vi "keyboard_monitor.vi"() -> ()   [LabVIEW 2019]
uses:
  <vilib>/Utility/inputDevices.llb/keyboardAcquire.vi
panel:
  out "error out":errorcluster
  out "handle out":i32
  in  "step":dbl
  in  "error in (no error)":errorcluster
  in  "handle in":i32
  in  "Up":bool
  in  "Down":bool
  in  "^":bool
  in  "v":bool
  in  ">":bool
  in  "<":bool
  out "x":dbl
  out "y":dbl
  out "z":dbl
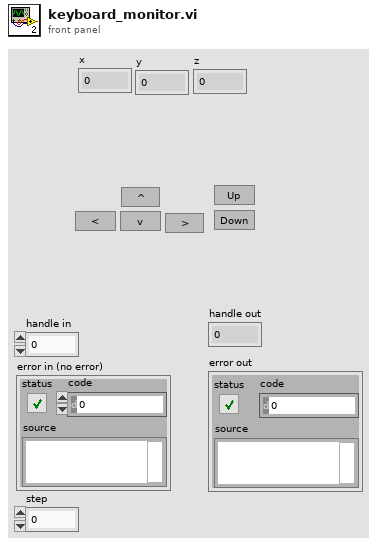
[diagram p1: front panel]
types:
  T1 = enum16{"0", "1", "2", "3", "4", "5", "6", "7", "8", "9", "A", "B", "C", "D", "E", "F", "G", "H", "I", "J", "K", "L", "M", "N", "O", "P", "Q", "R", "S", "T", "U", "V", "W", "X", "Y", "Z", "F1", "F2", "F3", "F4", "F5", "F6", "F7", "F8", "F9", "F10", "F11", "F12", "F13", "F14", "F15", "ADD", "BACK", "BACKSLASH", "CAPITAL", "COMMA", "DECIMAL", "DELETE", "DIVIDE", "DOWN", "END", "EQUALS", "ESCAPE", "GRAVE (`)", "HOME", "INSERT", "LBRACKET", "LCONTROL", "LEFT", "L ALT", "LSHIFT", "LWIN", "MINUS", "MULTIPLY", "NEXT", "NUMLOCK", "NUMPAD_0", "NUMPAD_1", "NUMPAD_2", "NUMPAD_3", "NUMPAD_4", "NUMPAD_5", "NUMPAD_6", "NUMPAD_7", "NUMPAD_8", "NUMPAD_9", "PAUSE", "PERIOD", "PRIOR (PG UP)", "RBRACKET", "RCONTROL", "RETURN", "RIGHT", "R ALT", "RSHIFT", "RWIN", "SCROLL", "SEMICOLON", "SLASH", "SPACE", "SUBTRACT", "TAB", "UP", "ENTER (num pad)", "' (quote)"}[]
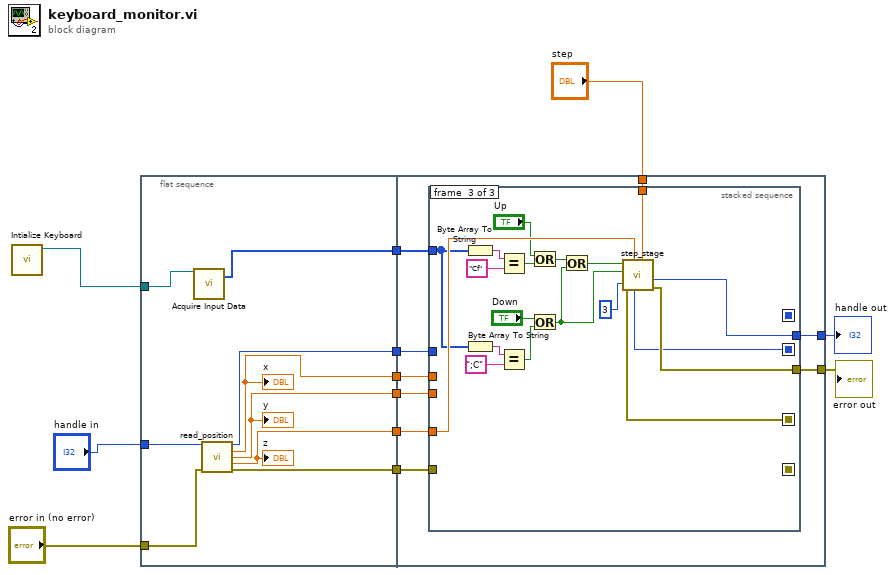
[diagram p0: block diagram]
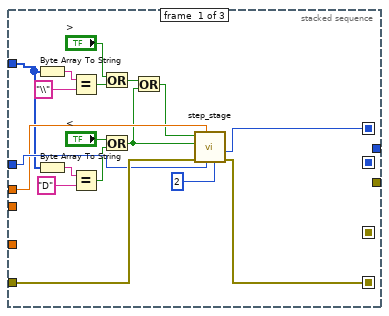
[diagram p2: hidden frame]
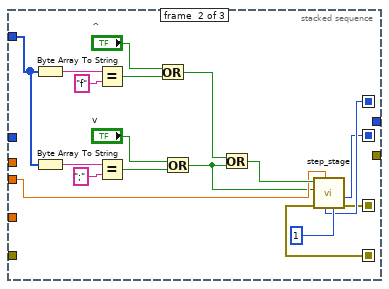
[diagram p3: hidden frame]
diagram:
  n1 = call <vilib>:"Intialize Keyboard.vi"() -> ("device ID"=w7:refnum<k1>)  [unwired: 1 in, 10 out]
  n2 = flat-sequence {
    tunnel: [w21] -> w12
    tunnel: [w20] -> w11
    tunnel: [w19] -> w10
    tunnel: [w18] -> w9
    tunnel: [w17] -> w8
    tunnel: w7 -> [w16]
    tunnel: [w15] -> w6
    tunnel: "handle in" -> [w14]
    tunnel: "error in (no error)" -> [w13]
    tunnel: w12 -> [w30]
    tunnel: w11 -> [w29]
    tunnel: w10 -> [w28]
    tunnel: w9 -> [w27]
    tunnel: w8 -> [w26]
    tunnel: [w25] -> w1
    tunnel: [w24] -> w2
    tunnel: w6 -> [w23]
    tunnel: "step" -> [w22]
    frame #0 {
      n3 = call-poly <vilib>:"Acquire Input Data.vi"("device ID"=w16) -> ("keys pressed"=w15:T1)  [unwired: 1 in, 17 out]
      n4 = call "read_position.vi"("handle in"=w14, "error in (no error)"=w13) -> ("handle out"=w20:i32, "x"=w19:dbl, "y"=w18:dbl, "z"=w17:dbl, "error out"=w21:errorcluster)  [unwired: 9 in]
      "x" <- w19
      "y" <- w18
      "z" <- w17
    }
    frame #1 {
      n5 = stacked-sequence {
        seq-local: [w44 _ _] -> [_ w63 _]
        seq-local: [w43 _ _] -> [_ w62 _]
        seq-local: [_ w60 _] -> [_ _ w81]
        seq-local: [_ w61 _] -> [_ _ w80]
        tunnel: w30 -> [w48 _ _]
        tunnel: w29 -> [w47 _ _]
        tunnel: w28 -> [w45 _ _]
        tunnel: w27 -> [_ w64 _]
        tunnel: w26 -> [_ _ w84]
        tunnel: [_ _ w82] -> w25
        tunnel: [_ _ w83] -> w24
        tunnel: w23 -> [w31 w49 w68]
        tunnel: w22 -> [_ _ w67]
        frame #0 {
          n6 = Byte Array To String(unsigned byte array=w31) -> (string=w42:string)
          n7 = Byte Array To String(unsigned byte array=w31) -> (string=w40:string)
          n8 = Equal?(x=w42, y="\\") -> (x = y?=w38:bool)
          n9 = Equal?(x=w40, y="D") -> (x = y?=w37:bool)
          n10 = Or(x=">", y=w38) -> (x .or. y?=w36:bool)
          n11 = Or(x="<", y=w37) -> (x .or. y?=w33:bool)
          n12 = Or(x=w36, y=w33) -> (x .or. y?=w32:bool)
          n13 = call "step_stage.vi"("axis"=u32 2, "handle"=w47, "position"=w45, "error in"=w48, "+/-"=w33, "move"=w32) -> ("error out"=w43:errorcluster, "handle out"=w44:i32)  [unwired: 4 in]
        }
        frame #1 {
          n14 = Byte Array To String(unsigned byte array=w49) -> (string=w59:string)
          n15 = Byte Array To String(unsigned byte array=w49) -> (string=w57:string)
          n16 = Equal?(x=w59, y="f") -> (x = y?=w55:bool)
          n17 = Equal?(x=w57, y=";") -> (x = y?=w52:bool)
          n18 = Or(x="^", y=w55) -> (x .or. y?=w51:bool)
          n19 = Or(x="v", y=w52) -> (x .or. y?=w50:bool)
          n20 = Or(x=w51, y=w50) -> (x .or. y?=w66:bool)
          n21 = call "step_stage.vi"("axis"=u32 1, "handle"=w63, "position"=w64, "error in"=w62, "+/-"=w50, "move"=w66) -> ("error out"=w61:errorcluster, "handle out"=w60:i32)  [unwired: 4 in]
        }
        frame #2 {
          n22 = Byte Array To String(unsigned byte array=w68) -> (string=w79:string)
          n23 = Byte Array To String(unsigned byte array=w68) -> (string=w77:string)
          n24 = Equal?(x=w79, y="Cf") -> (x = y?=w75:bool)
          n25 = Equal?(x=w77, y=";C") -> (x = y?=w74:bool)
          n26 = Or(x="Up", y=w75) -> (x .or. y?=w73:bool)
          n27 = Or(x="Down", y=w74) -> (x .or. y?=w71:bool)
          n28 = Or(x=w73, y=w71) -> (x .or. y?=w72:bool)
          n29 = call "step_stage.vi"("axis"=u32 3, "step"=w67, "handle"=w81, "position"=w84, "error in"=w80, "+/-"=w71, "move"=w72) -> ("error out"=w82:errorcluster, "handle out"=w83:i32)  [unwired: 3 in]
        }
      }
    }
  }
  "handle out" <- w2
  "error out" <- w1
